vi "MQTT_Read_Published_Message.vi"(8 "error in (no error)":errorcluster, 11 "connection ID":refnum<k5>) -> (0 "error out":errorcluster, 1 "Message":string="MQIsdp", 2 "Topic Name":string="Topic", 3 "connection ID out":refnum<k5>, 4 "MessageType":T1, 5 "Message ID":u16=1 format="%x")   [LabVIEW 2012, in "MQTT_Functions.lvlib"]
uses:
  MQTT_Functions.lvlib
  Controls/MessageType.ctl
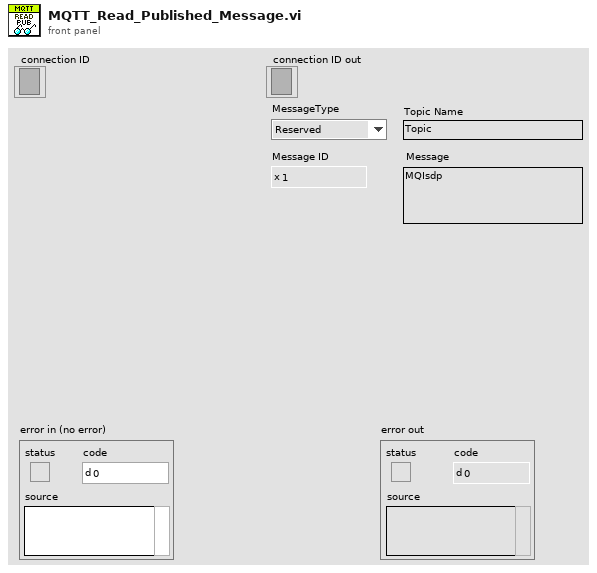
[diagram p1: front panel]
types:
  T1 = typedef "MQTT_Functions.lvlib/MessageType.ctl" = enum32{"Reserved", "CONNECT", "CONNACK", "PUBLISH", "PUBACK", "PUBREC", "PUBREL", "PUBCOMP", "SUBSCRIBE", "SUBACK", "UNSUBSCRIBE", "UNSUBACK", "PINGREQ", "PINGRESP", "DISCONNECT", "Reserved2"}
  T2 = typedef "MQTT_Functions.lvlib/QoS.ctl" = enum8{"At most once", "At least once", "Exactly once", "Reserved"}
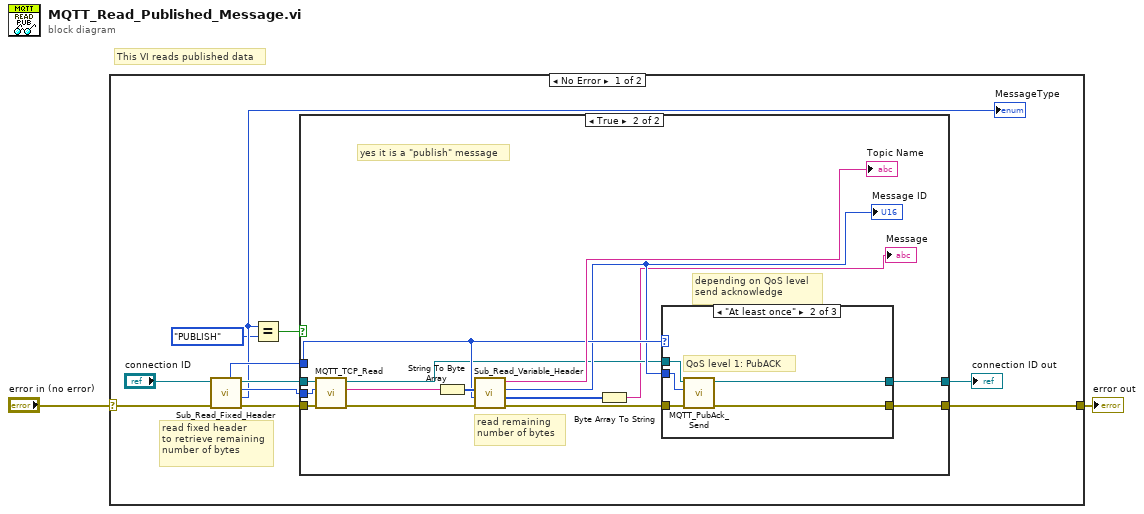
[diagram p0: block diagram]
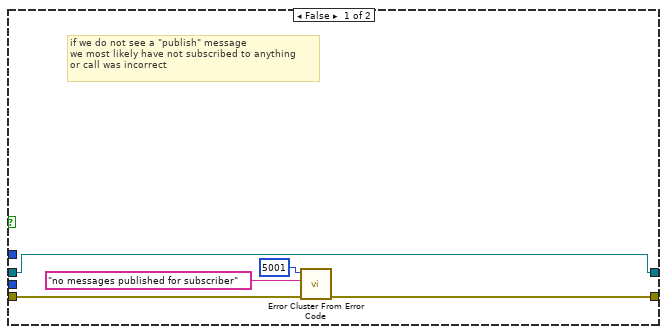
[diagram p2: hidden frame]
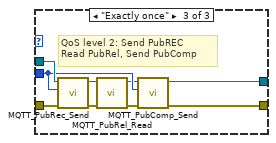
[diagram p4: hidden frame]
diagram:
  # "This VI reads published data"
  n1 = case shown="No Error" "error in (no error)" {
    selector: "error in (no error)" -> [w12 w50]
    tunnel: [w6 w50] -> w1
    frame No Error {
      # "read fixed header \nto retrieve remaining\nnumber of bytes"
      n2 = call "Sub_Read_Fixed_Header.vi"("error in (no error)"=w12, "connection ID"="connection ID") -> ("error out"=w9:errorcluster, "MessageType"=w5:T1, "Remaining Length"=w11:u32, "connection ID out"=w10:refnum<k5>, "QoS Level"=w8:T2)  [unwired: 3 in, 2 out]
      "MessageType" <- w5
      n3 = Equal?(x=w5, y=MessageType."PUBLISH") -> (x = y?=w3:bool)
      n4 = case shown="True" w3 {
        tunnel: w11 -> [_ w32]
        tunnel: w10 -> [w14 w31]
        tunnel: w9 -> [w18 w30]
        tunnel: w8 -> [_ w26]
        tunnel: [w14 w23] -> w7
        tunnel: [w15 w22] -> w6
        frame False {
          # "if we do not see a \"publish\" message\nwe most likely have not subscribed to anything\nor call was incorrect"
          n5 = call <vilib>:"Error Cluster From Error Code.vi"("error in (no error)"=w18, "error message (\"\")"="no messages published for subscriber" ("error message (\"\")"), "error code (0)"=5001) -> ("error out"=w15:errorcluster)  [unwired: 6 in]
        }
        frame True {
          # "yes it is a \"publish\" message"
          # "depending on QoS level\nsend acknowledge"
          # "read remaining\nnumber of bytes"
          n6 = call "MQTT_TCP_Read.vi"("error in (no error)"=w30, "bytes to read"=w32, "connection ID"=w31) -> ("error out"=w27:errorcluster, "data out"=w29:string, "connection ID out"=w24:refnum<k5>)  [unwired: 6 in]
          n7 = String To Byte Array(string=w29) -> (unsigned byte array=w28:u8[])
          n8 = call "Sub_Read_Variable_Header.vi"("error in (no error)"=w27, "QoS"=w26, "Variable Header"=w28) -> ("error out"=w21:errorcluster, "remaining bytes"=w19:u8[], "Message ID"=w25:u16, "Topic Name"=→"Topic Name":string)  [unwired: 5 in]
          "Message ID" <- w25
          n9 = Byte Array To String(unsigned byte array=w19) -> (string=→"Message":string)
          n10 = case shown="\"At least once\"" w26 {
            tunnel: w25 -> [_ w40 w45]
            tunnel: w21 -> [w34 w39 w49]
            tunnel: w24 -> [w35 w38 w48]
            tunnel: [w35 w37 w47] -> w23
            tunnel: [w34 w36 w46] -> w22
            frame "At most once", Default {
              # "QoS level 0, no ACK"
            }
            frame "At least once" {
              # "QoS level 1: PubACK"
              n11 = call "MQTT_PubAck_Send.vi"("error in (no error)"=w39, "Message ID"=w40, "connection ID"=w38) -> ("error out"=w36:errorcluster, "connection ID out"=w37:refnum<k5>)  [unwired: 6 in, 1 out]
            }
            frame "Exactly once" {
              # "QoS level 2: Send PubREC\nRead PubRel, Send PubComp"
              n12 = call "MQTT_PubRec_Send.vi"("error in (no error)"=w49, "Message ID"=w45, "connection ID"=w48) -> ("error out"=w42:errorcluster, "connection ID out"=w41:refnum<k5>)  [unwired: 6 in, 1 out]
              n13 = call "MQTT_PubRel_Read.vi"("error in (no error)"=w42, "connection ID"=w41) -> ("error out"=w43:errorcluster, "connection ID out"=w44:refnum<k5>)  [unwired: 7 in, 1 out]
              n14 = call "MQTT_PubComp_Send.vi"("error in (no error)"=w43, "Message ID"=w45, "connection ID"=w44) -> ("error out"=w46:errorcluster, "connection ID out"=w47:refnum<k5>)  [unwired: 6 in, 1 out]
            }
          }
        }
      }
      "connection ID out" <- w7
    }
    frame Error {
    }
  }
  "error out" <- w1
